vi "Water Tank.vi"() -> ()   [LabVIEW 2013]
uses:
  Water Tank Global.vi
panel:
  in  "Manual Control":bool
  out "Bottom Float Switch":bool
  out "Top Float Switch":bool
  out "Water level":i32(slide) scale=0.0..300.0
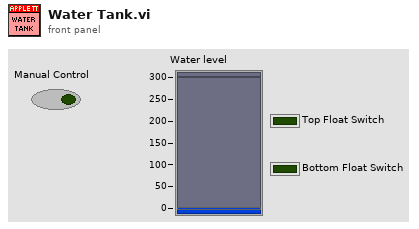
[diagram p1: front panel]
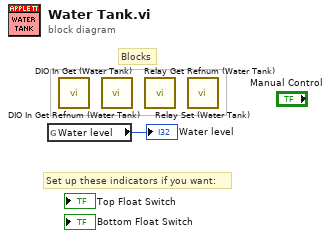
[diagram p0: block diagram]
diagram:
  # "Set up these indicators if you want:"
  # "Blocks"
  n1 = global read "Water Tank Global.vi" "Water level"() -> (→"Water level":i32)
  n2 = call "DIO In Get Refnum (Water Tank).vi"() -> ()  [unwired: 10 in, 2 out]
  n3 = call "DIO In Get (Water Tank).vi"() -> ()  [unwired: 9 in, 3 out]
  n4 = call "Relay Get Refnum (Water Tank).vi"() -> ()  [unwired: 10 in, 2 out]
  n5 = call "Relay Set (Water Tank).vi"() -> ()  [unwired: 10 in, 2 out]
